vi "dvp Vi Set Ae Mode.vi"(10 "AeMode":u32(ring) items=["AE_MODE_AE_AG", "AE_MODE_AG_AE", "AE_MODE_AE_ONLY", "AE_MODE_AG_ONLY"], 11 "handle":u32) -> (3 "function return":u32(ring))   [LabVIEW 2018, in "LabViewDVPCamera.lvlib"]
doc: "LabviewDvp2Api dvpStatus dvpViSetAeMode(dvpHandle handle, dvpAeMode AeMode);"
uses:
  LabViewDVPCamera.lvlib
  LabViewDVPCamera/LabViewDVPCamera.dll
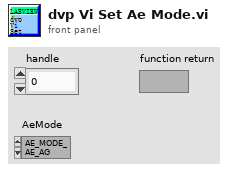
[diagram p1: front panel]
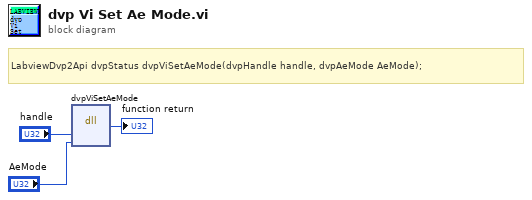
[diagram p0: block diagram]
diagram:
  # "LabviewDvp2Api dvpStatus dvpViSetAeMode(dvpHandle handle, dvpAeMode AeMode);"
  n1 = dll-call lib="C:/Program Files (x86)/DVP2 Labview cn 64/Sample/LabViewDVPCamera/LabViewDVPCamera.*" fn="dvpViSetAeMode"("handle"="handle", "AeMode"="AeMode") -> (→"function return":u32)  [unwired: 5 in, 2 out]
